vi "Send REM Command.vi"(8 "error in (no error)":errorcluster, 11 "Switch Program":T1) -> (0 "error out":errorcluster)   [LabVIEW 2014]
doc: "Sends the REM command. This tells the myRIO to remove a specific switch program."
uses:
  myRIO/Controls/Switch Program.ctl
  myRIO/Controls/Action Enum.ctl
  myRIO/Controls/Switch Day.ctl
  Controls/UDP Reference Action Enum.ctl
panel:
  out "concatenated string":string
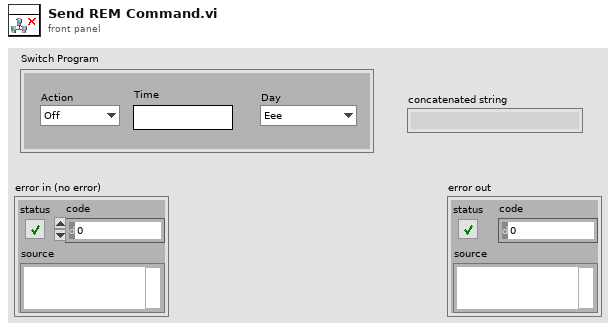
[diagram p1: front panel]
types:
  T1 = typedef "Switch Program.ctl" = cluster{"Action":T2, "Time":string, "Day":T3}
  T2 = typedef "Action Enum.ctl" = enum16{"Off", "On"}
  T3 = typedef "Switch Day.ctl" = enum16{"Eee", "Sun", "Mon", "Tue", "Wed", "Thu", "Fri", "Sat"}
  T4 = typedef "UDP Reference Action Enum.ctl" = enum16{"Set", "Get"}
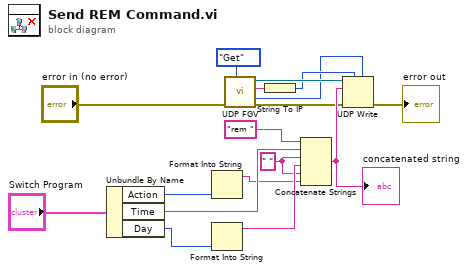
[diagram p0: block diagram]
diagram:
  w2 = " "
  n1 = Unbundle By Name("Switch Program") -> ("Action"=w6:T2, "Time"=w4:string, "Day"=w5:T3)
  n2 = Format Into String(w6) -> (resulting string=w1:string)  [unwired: 3 in, 1 out]
  n3 = Format Into String(w5) -> (resulting string=w3:string)  [unwired: 3 in, 1 out]
  n4 = call "UDP FGV.vi"("Action"=UDP_Reference_Action_Enum."Get", "error in (no error)"="error in (no error)") -> ("error out"=w13:errorcluster, "Port Out"=w8:u16, "IP Address out"=w10:string, "connection ID out"=w14:refnum<k16>)  [unwired: 6 in]
  n5 = String To IP(1:w10) -> (0:w9:u32)
  n6 = Concatenate Strings("rem ", w4, w2, w3, w2, w1) -> (w17:string)
  "concatenated string" <- w17
  n7 = UDP Write(address=w9, port or service name=w8, connection ID=w14, data in=w17, 8:w13) -> (error out=→"error out":errorcluster)  [unwired: 1 in, 1 out]
